vi "Fetch FPGA Data.vi"(0 "Register Bus":T2, 4 "Tx Constant":cluster{"cte I":i16, "cte Q":i16}, 5 "Beta":fxp<+,26,24>, 7 "error in":errorcluster, 8 "Select Wave":u8, 9 "vertical range [Vpp]":dbl=2.0 format="%#_6p", 12 "PRP (ms)":dbl, 13 "sample rate [S/s]":dbl=130000000.0 format="%#_6p", 14 "Pulse width (us)":dbl format="%#_10g", 15 "Guard width (us)":dbl format="%#_10g", 16 "Oversampling factor":u8, 17 "FPGA VI Reference In":refnum<k20>, 24 "nroCPI x CPI":u32, 25 "numRange":u32, 26 "pulseRange":u32) -> (20 "Register Bus (out)":T2, 21 "Rx Waveform (CDB WDT)":waveform(cdb), 23 "Tx Waveform (CDB WDT)":waveform(cdb), 27 "error out":errorcluster)   [LabVIEW 2017]
doc: "Fetch Rx data from the device. It's required to call <b>Configure Stream</b> and <b>Initiate Stream</b> before calling this VI."
uses:
  <instrlib>/_niInstr/Register Bus/v0/Host/Public/Register Bus Session.ctl
  <instrlib>/_niInstr/Register Bus/v0/Host/Private/Session Data.ctl
  <vilib>/Utility/error.llb/Error Cluster From Error Code.vi
  <vilib>/rvi/errors/niLvFpgaAdjustHostInterfaceError.vi
  <vilib>/Analysis/2dsp.llb/Rational Resample (single channel, DBL).vi
  <vilib>/rvi/interface/nirviReadWriteControl/nirviReadWriteControl.xnode
  <vilib>/rvi/interface/nirviMethod/nirviMethod.xnode
  <instrlib>/_niInstr/Register Bus/v0/Host/niInstr Register Bus v0 Host.lvlib
  <vilib>/FPGAPlugInAG/Dynamic/niLvFpga_ReadFifo_Dynamic.vi
  <vilib>/rvi/errors/niLvFpgaMergeErrorWithErrorCode.vi
  <vilib>/Analysis/NI_AALPro.lvlib
  NiFpgaLv.dll
  <vilib>/rvi/interface/Simulation/niFpgaSimulationCallBeginRW.vi
panel:
  in  "FIR filter specifications":T1={"alias rejection (dB)"=60.0, "normalized bandwidth"=0.42} {"normalized bandwidth" format="%#.6g"; "alias rejection (dB)" format="%#.6g"}
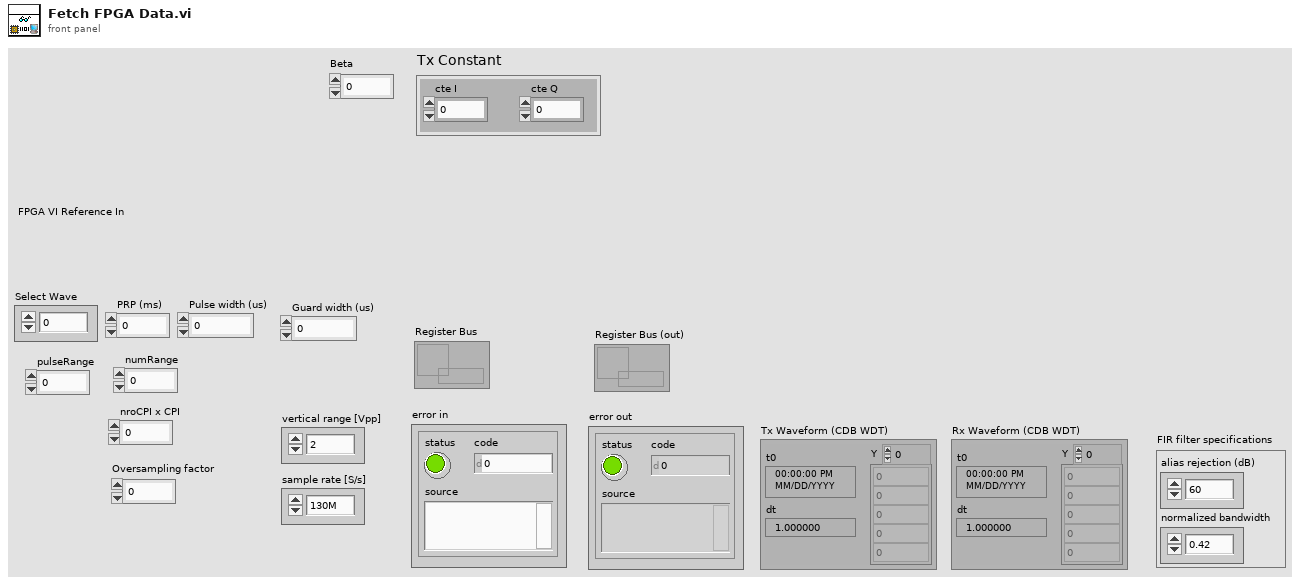
[diagram p1: front panel]
types:
  T1 = cluster{"alias rejection (dB)":dbl, "normalized bandwidth":dbl}
  T2 = typedef "niInstr Register Bus v0 Host.lvlib/Register Bus Session.ctl" = refnum<queue>
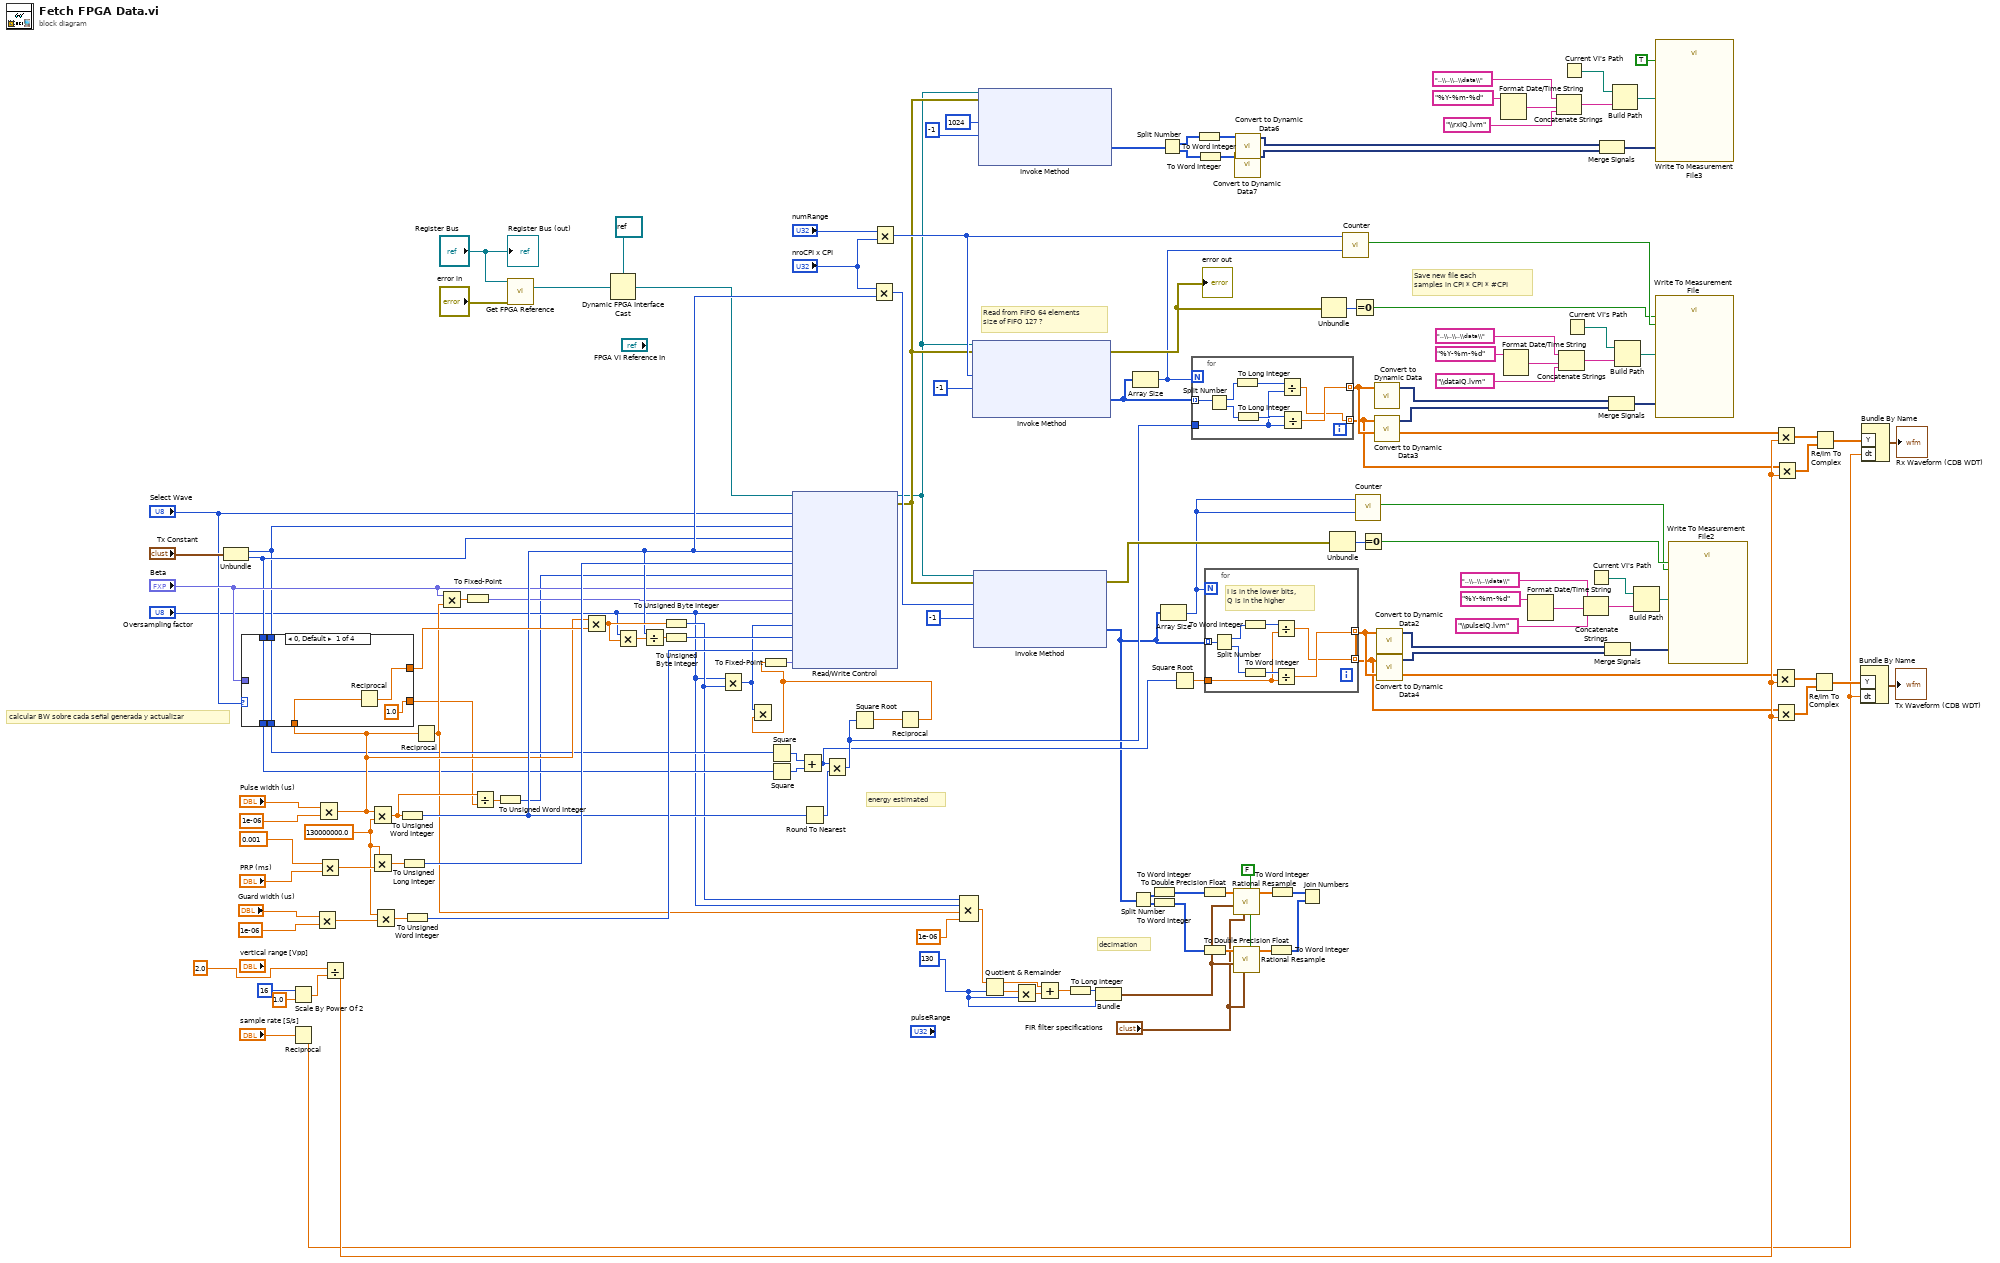
[diagram p0: block diagram]
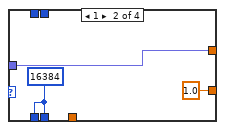
[diagram p2: hidden frame]
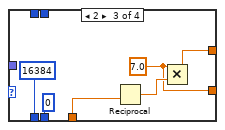
[diagram p3: hidden frame]
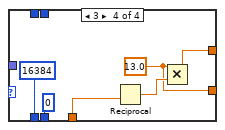
[diagram p4: hidden frame]
diagram:
  w51 = FALSE ("reset")
  w67 = 130
  w100 = 130000000.0
  # "decimation"
  # "energy estimated"
  # "Read from FIFO 64 elements\nsize of FIFO 127 ?"
  # "Save new file each \nsamples in CPI * CPI * #CPI"
  # "calcular BW sobre cada señal generada y actualizar"
  n1 = Unbundle("Tx Constant") -> ("cte I"=w43:i16, "cte Q"=w44:i16)
  n2 = Scale By Power Of 2(n=i16 16 ("ADC Resolution (bits)"), x=1.0) -> (x*2^n=w145:dbl)
  n3 = Reciprocal(x="sample rate [S/s]") -> (1/x=w108:dbl)
  n4 = Multiply(x="Guard width (us)", y=1e-06) -> (x*y=w101:dbl)
  n5 = Multiply(x="Pulse width (us)", y=1e-06) -> (x*y=w46:dbl)
  n6 = case shown="0, Default" "Select Wave" {
    tunnel: w46 -> [w154 _ w162 w168]
    tunnel: [w153 w157 w163 w169] -> w107
    tunnel: "Beta" -> [_ w157 _ _]
    tunnel: w44 -> [w152 _ _ _]
    tunnel: [w152 w156 16384 16384] -> w41
    tunnel: w43 -> [w151 _ _ _]
    tunnel: [w151 w156 i16 0 i16 0] -> w42
    tunnel: [1.0 ("y") 1.0 ("y") w158 w164] -> w38
    frame 0, Default {
      n7 = Reciprocal(x=w154) -> (1/x=w153:dbl)
    }
    frame 1 {
      w156 = 16384
    }
    frame 2 {
      w158 = 7.0 ("y")
      n8 = Reciprocal(x=w162) -> (1/x=w161:dbl)
      n9 = Multiply(x=w158, y=w161) -> (x*y=w163:dbl)
    }
    frame 3 {
      w164 = 13.0 ("y")
      n10 = Reciprocal(x=w168) -> (1/x=w167:dbl)
      n11 = Multiply(x=w164, y=w167) -> (x*y=w169:dbl)
    }
  }
  n12 = Multiply(x=0.001, y="PRP (ms)") -> (x*y=w105:dbl)
  n13 = Divide(x=2.0, y=w145) -> (x/y=w122:dbl)
  n14 = Multiply(x=w46, y=w100) -> (x*y=w135:dbl)
  n15 = Multiply(x=w100, y=w105) -> (x*y=w137:dbl)
  n16 = Multiply(x=w100, y=w101) -> (x*y=w102:dbl)
  n17 = To Unsigned Word Integer(number=w135) -> (unsigned 16bit integer=w65:u16)
  n18 = To Unsigned Long Integer(number=w137) -> (unsigned 32bit integer=w109:u32)
  n19 = To Unsigned Word Integer(number=w102) -> (unsigned 16bit integer=w99:u16)
  n20 = Reciprocal(x=w46) -> (1/x=w45:dbl)
  n21 = Multiply(x="Beta", y=w45) -> (x*y=w49:dbl)
  n22 = To Fixed-Point(number=w49) -> (fixed-point=w47:fxp<+,52,48>)  [unwired: 1 in]
  n23 = Divide(x=w135, y=w38) -> (x/y=w136:dbl)
  n24 = To Unsigned Word Integer(number=w136) -> (unsigned 16bit integer=w26:u16)
  n25 = call <instrlib>:"Get FPGA Reference.vi"("session in"="Register Bus", "error in"="error in") -> ("fpga ref"=w139:refnum<k20>)  [unwired: 11 in, 2 out]
  n26 = Multiply(x=w46, y=w107) -> (x*y=w110:dbl)
  n27 = Dynamic FPGA Interface Cast(Session In=refnum<k20> refnum ("FPGA Interface"), Type=w139) -> (Session Out=w1:refnum<k20>)
  n28 = Multiply(x="Oversampling factor", y=w110) -> (x*y=w112:dbl)
  n29 = Divide(x=w65, y=w112) -> (x/y=w111:dbl)
  n30 = To Unsigned Byte Integer(number=w110) -> (unsigned 8bit integer=w36:u8)
  n31 = To Unsigned Byte Integer(number=w111) -> (unsigned 8bit integer=w98:u8)
  n32 = Multiply(x="Oversampling factor", y=w36) -> (x*y=w34:u8)
  n33 = Square(x=w42) -> (x^2=w90:u64)
  n34 = Square(x=w41) -> (x^2=w91:u64)
  n35 = Add(x=w90, y=w91) -> (x+y=w29:u64)
  n36 = Round To Nearest(number=w65) -> (nearest integer value=w89:u16)
  n37 = Multiply(x=w29, y=w89) -> (x*y=w30:u64)
  n38 = Square Root(x=w30) -> (sqrt(x)=w32:dbl)
  n39 = Multiply(x="nroCPI x CPI", y=w65) -> (x*y=w64:u32)
  n40 = Multiply(x="numRange", y="nroCPI x CPI") -> (x*y=w25:u32)
  n41 = Reciprocal(x=w32) -> (1/x=w31:dbl)
  n42 = Multiply(x=w34, y=w31) -> ()  [unwired: 1 out]
  n43 = To Fixed-Point(number=w31) -> (fixed-point=w33:fxp<+,48,0>)  [unwired: 1 in]
  n44 = xnode "Read/Write Control"("FPGA VI Reference In"=w1, "Select Wave"="Select Wave", "cte I"=w43, "cte Q"=w44, "Pulse width"=w65, "PRP"=w109, "Chip width"=w26, "Beta"="Beta", "Beta/tao"=w47, "Oversampling factor"="Oversampling factor", "N"=w34, "Delta"=w98, "Guard width"=w99, "Pulse Energy"=w33) -> ("FPGA VI Reference Out"=w22:refnum<k20>, "error out"=w23:errorcluster)  [unwired: 1 in]
  n45 = Compound Arithmetic op=MULTIPLY(w36, "Oversampling factor", w45, 1e-06) -> (w72:dbl)
  n46 = xnode "Invoke Method"("FPGA VI Reference In"=w22, "error in"=w23, "Number of Elements"=w25, "Timeout (ms)"=-1) -> ("error out"=w116:errorcluster, "Data"=w93:u64[])  [unwired: 2 out]
  "error out" <- w116
  n47 = xnode "Invoke Method"("FPGA VI Reference In"=w22, "error in"=w23, "Number of Elements"=w64, "Timeout (ms)"=-1) -> ("error out"=w114:errorcluster, "Data"=w27:u32[])  [unwired: 2 out]
  n48 = xnode "Invoke Method"("FPGA VI Reference In"=w22, "error in"=w23, "Number of Elements"=u32 1024, "Timeout (ms)"=-1) -> ("Data"=w10:u32[])  [unwired: 3 out]
  n49 = Quotient & Remainder(x=w72, y=w67) -> (x-y*floor(x/y)=w70:dbl, floor(x/y)=w69:dbl)
  n50 = Multiply(x=w69, y=w67) -> (x*y=w71:dbl)
  n51 = Add(x=w70, y=w71) -> (x+y=w68:dbl)
  n52 = To Long Integer(number=w68) -> (32bit integer=w73:i32)
  n53 = Bundle(w73, w67) -> (w58:cluster{i32, i32})  [unwired: 1 in]
  n54 = Split Number(x=w27) -> (hi(x)=w63:u16[], lo(x)=w62:u16[])
  n55 = Array Size(array=w93) -> (size(s)=w12:i32)
  n56 = To Word Integer(number=w63) -> (16bit integer=w61:i16[])
  n57 = To Word Integer(number=w62) -> (16bit integer=w59:i16[])
  n58 = Split Number(x=w10) -> (hi(x)=w5:u16[], lo(x)=w4:u16[])
  n59 = Array Size(array=w27) -> (size(s)=w52:i32)
  n60 = Square Root(x=w29) -> (sqrt(x)=w28:dbl)
  n61 = for {
    N: w12 -> [_]
    tunnel: w93 -> [w175] mode=indexing
    tunnel: [w171] -> w40 mode=indexing
    tunnel: [w170] -> w39 mode=indexing
    tunnel: w30 -> [w172]
    n62 = Split Number(x=w175) -> (hi(x)=w177:u32, lo(x)=w176:u32)
    n63 = To Long Integer(number=w177) -> (32bit integer=w174:i32)
    n64 = To Long Integer(number=w176) -> (32bit integer=w173:i32)
    n65 = Divide(x=w174, y=w172) -> (x/y=w170:dbl)
    n66 = Divide(x=w173, y=w172) -> (x/y=w171:dbl)
  }
  n67 = To Word Integer(number=w5) -> (16bit integer=w6:i16[])
  n68 = To Word Integer(number=w4) -> (16bit integer=w3:i16[])
  n69 = To Double Precision Float(number=w61) -> (double precision float=w74:dbl[])
  n70 = To Double Precision Float(number=w59) -> (double precision float=w60:dbl[])
  n71 = for {
    N: w52 -> [_]
    tunnel: [w178] -> w77 mode=indexing
    tunnel: [w181] -> w78 mode=indexing
    tunnel: w27 -> [w183] mode=indexing
    tunnel: w28 -> [w179]
    # "I is in the lower bits,\nQ is in the higher"
    n72 = Split Number(x=w183) -> (hi(x)=w185:u16, lo(x)=w184:u16)
    n73 = To Word Integer(number=w185) -> (16bit integer=w180:i16)
    n74 = To Word Integer(number=w184) -> (16bit integer=w182:i16)
    n75 = Divide(x=w180, y=w179) -> (x/y=w178:dbl)
    n76 = Divide(x=w182, y=w179) -> (x/y=w181:dbl)
  }
  n77 = call-poly <vilib>:"Rational Resample.vi"("anti-aliasing?"=w51, "FIR filter specifications"="FIR filter specifications", "resample factor"=w58, "X"=w74) -> ("Y"=w57:dbl[])  [unwired: 5 in, 2 out]
  n78 = call-poly <vilib>:"Rational Resample.vi"("anti-aliasing?"=w51, "FIR filter specifications"="FIR filter specifications", "resample factor"=w58, "X"=w60) -> ("Y"=w56:dbl[])  [unwired: 5 in, 2 out]
  n79 = call "Convert to Dynamic Data7"("Array"=w3) -> ("Dynamic Data Type"=w8:dynamicdata)  [unwired: 3 in]
  n80 = call "Convert to Dynamic Data6"("Array"=w6) -> ("Dynamic Data Type"=w7:dynamicdata)  [unwired: 3 in]
  n81 = To Word Integer(number=w56) -> (16bit integer=w54:i16[])
  n82 = To Word Integer(number=w57) -> (16bit integer=w55:i16[])
  n83 = Join Numbers(hi=w55, lo=w54) -> ()  [unwired: 1 out]
  n84 = Unbundle(w116) -> ("code"=w117:i32)  [unwired: 2 out]
  n85 = Unbundle(w114) -> ("code"=w115:i32)  [unwired: 2 out]
  n86 = call "Counter.vi"("step"=w12, "limit"=w25) -> ("count = limit?"=w14:bool)  [unwired: 8 in, 1 out]
  n87 = Equal To 0?(x=w117) -> (x = 0?=w13:bool)
  n88 = call "Counter.vi"("step"=w52, "limit"=w52) -> ("count = limit?"=w76:bool)  [unwired: 8 in, 1 out]
  n89 = Equal To 0?(x=w115) -> (x = 0?=w113:bool)
  n90 = call "Convert to Dynamic Data"("Array"=w40) -> ("Dynamic Data Type"=w106:dynamicdata)  [unwired: 3 in]
  n91 = call "Convert to Dynamic Data3"("Array"=w39) -> ("Dynamic Data Type"=w121:dynamicdata)  [unwired: 3 in]
  n92 = call "Convert to Dynamic Data2"("Array"=w78) -> ("Dynamic Data Type"=w120:dynamicdata)  [unwired: 3 in]
  n93 = call "Convert to Dynamic Data4"("Array"=w77) -> ("Dynamic Data Type"=w119:dynamicdata)  [unwired: 3 in]
  n94 = Format Date/Time String(time format string (%c)="%Y-%m-%d") -> (date/time string=w18:string)  [unwired: 2 in]
  n95 = Format Date/Time String(time format string (%c)="%Y-%m-%d") -> (date/time string=w87:string)  [unwired: 2 in]
  n96 = Format Date/Time String(time format string (%c)="%Y-%m-%d") -> (date/time string=w82:string)  [unwired: 2 in]
  n97 = Concatenate Strings("..\\..\\..\\data\\" ("name or relative path"), w18, "\\rxIQ.lvm" ("name or relative path")) -> (w15:string)
  n98 = Concatenate Strings("..\\..\\..\\data\\" ("name or relative path"), w87, "\\dataIQ.lvm" ("name or relative path")) -> (w84:string)
  n99 = Current VI's Path() -> (path=w21:path)
  n100 = Current VI's Path() -> (path=w97:path)
  n101 = Concatenate Strings("..\\..\\..\\data\\" ("name or relative path"), w82, "\\pulseIQ.lvm" ("name or relative path")) -> (w79:string)
  n102 = Current VI's Path() -> (path=w95:path)
  n103 = Merge Signals(w7, w8) -> (w9:dynamicdata)
  n104 = Merge Signals(w120, w119) -> (w118:dynamicdata)
  n105 = Merge Signals(w106, w121) -> (w92:dynamicdata)
  n106 = Build Path(base path=w21, name or relative path=w15) -> (appended path=w20:path)
  n107 = Build Path(base path=w97, name or relative path=w84) -> (appended path=w96:path)
  n108 = Build Path(base path=w95, name or relative path=w79) -> (appended path=w94:path)
  n109 = call "Write To Measurement File3"("Signals"=w9, "Enable"=TRUE, "Filename"=w20) -> ()  [unwired: 14 in, 3 out]
  n110 = call "Write To Measurement File"("Signals"=w92, "Enable"=w13, "new_file"=w14, "Filename"=w96) -> ()  [unwired: 13 in, 3 out]
  n111 = call "Write To Measurement File2"("Signals"=w118, "Enable"=w113, "new_file"=w76, "Filename"=w94) -> ()  [unwired: 13 in, 3 out]
  n112 = Multiply(x=w78, y=w122) -> (x*y=w124:dbl[])
  n113 = Multiply(x=w40, y=w122) -> (x*y=w144:dbl[])
  n114 = Multiply(x=w77, y=w122) -> (x*y=w125:dbl[])
  n115 = Multiply(x=w39, y=w122) -> (x*y=w143:dbl[])
  n116 = Re/Im To Complex(1:w125, 2:w124) -> (0:w126:cdb[])
  n117 = Re/Im To Complex(1:w143, 2:w144) -> (0:w142:cdb[])
  n118 = Bundle By Name("Y"=w126, "dt"=w108) -> (→"Tx Waveform (CDB WDT)":waveform(cdb))  [unwired: 1 in]
  n119 = Bundle By Name("Y"=w142, "dt"=w108) -> (→"Rx Waveform (CDB WDT)":waveform(cdb))  [unwired: 1 in]
  "Register Bus (out)" <- "Register Bus"
